vi "Make Data Point.vi"(4 "Add Data Point (F)":bool, 6 "Data Log Indicies":i32[](array[numeric]), 7 "Samples Recorded":u32, 9 "Data":sgl[](array[numeric]), 10 "Array in":string[][](array[string]), 11 "Start Time":timestamp) -> (2 "Array out":string[][](array[string]), 3 "Samples Recorded":u32)   [LabVIEW 2023]
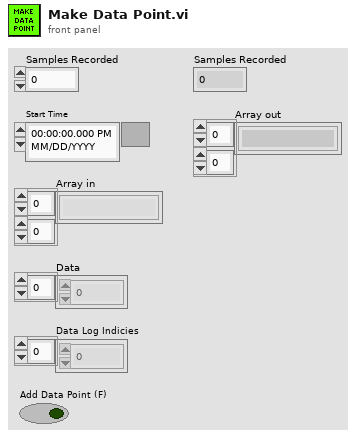
[diagram p1: front panel]
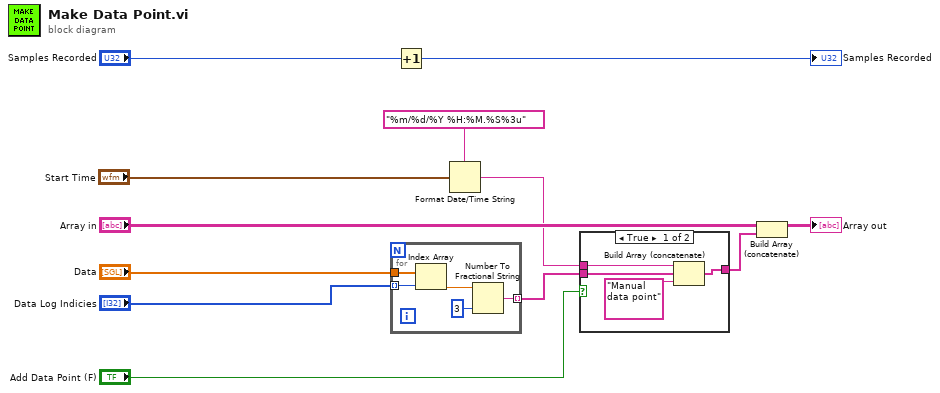
[diagram p0: block diagram]
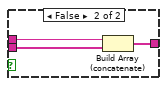
[diagram p2: hidden frame]
diagram:
  n1 = for {
    tunnel: "Data" -> [w17]
    tunnel: "Data Log Indicies" -> [w16] mode=indexing
    tunnel: [w13] -> w3 mode=indexing
    n2 = Index Array(array=w17, index=w16) -> (element=w15:sgl)
    n3 = Number To Fractional String(number=w15, precision (6)=i16 3) -> (F-format string=w13:string)  [unwired: 2 in]
  }
  n4 = Increment(x="Samples Recorded") -> (x+1=→"Samples Recorded":u32)
  n5 = Format Date/Time String(time format string (%c)="%m/%d/%Y %H:%M.%S%3u", seconds (now)="Start Time") -> (date/time string=w4:string)  [unwired: 1 in]
  n6 = case shown="True" "Add Data Point (F)" {
    tunnel: w3 -> [w21 w24]
    tunnel: w4 -> [w18 w23]
    tunnel: [w20 w22] -> w5
    frame True {
      n7 = Build Array (concatenate)(w18, w21, "Manual data point") -> (w20:string[])
    }
    frame False {
      n8 = Build Array (concatenate)(w23, w24) -> (w22:string[])
    }
  }
  n9 = Build Array (concatenate)("Array in", w5) -> (→"Array out":string[][])
